vi "filter.delete.order.vi"(11 "filter.data in":T1 {"memory.command"."order.slot.value"."Quantity" format="%016x"; "memory.command"."order.slot.value"."OrderId" format="%016x"; "memory.command"."ticker.slot.value"."Symbol" format="%016x"; "Scratch"."OrderId" format="%016x"}) -> (3 "filter.data out":T1 {"memory.command"."order.slot.value"."Quantity" format="%016x"; "memory.command"."order.slot.value"."OrderId" format="%016x"; "memory.command"."ticker.slot.value"."Symbol" format="%016x"; "Scratch"."OrderId" format="%016x"})   [LabVIEW 2022 SP3]
uses:
  filter.data.ctl
  filter.states.ctl
  filter.debug.ctl
  filter.debug.slot.ctl
  filter.data.scratch.ctl
  common/orderbook.command.ctl
  common/orderbook.command.type.ctl
  filter.memory.command.ctl
  ticker.slot.ctl
  order.slot.ctl
  filter.getstate.ctl
  filter.getstate.slot.ctl
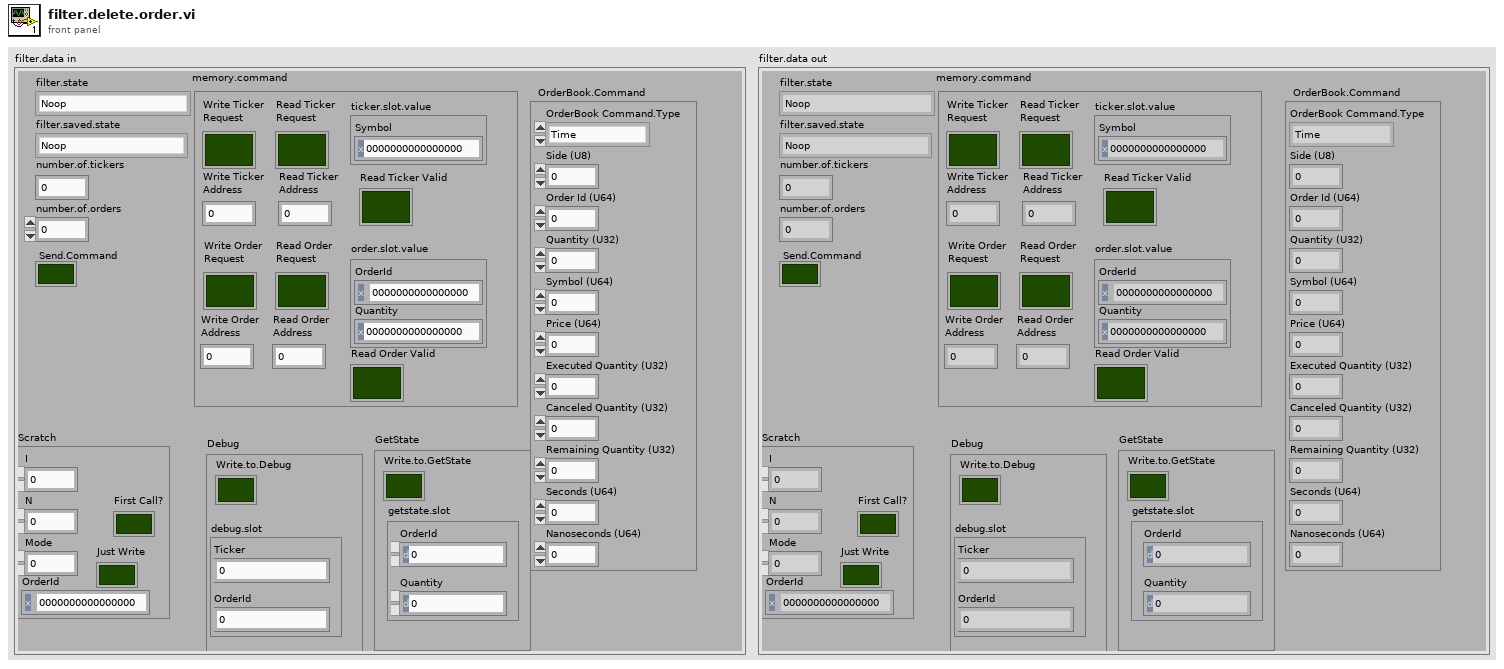
[diagram p1: front panel]
types:
  T1 = typedef "filter.data.ctl" = cluster{"filter.state":T2, "Debug":T3, "number.of.tickers":u32, "number.of.orders":u32, "filter.saved.state":T2, "Scratch":T5, "OrderBook.Command":T6, "Send.Command":bool, "memory.command":T8, "GetState":T11}
  T2 = typedef "filter.states.ctl" = enum16{"Noop", "Reset", "Debug", "Configuration", "Get.State", "Wait.for.Command", "Filter.Add", "Filter.Other", "Insert.Order", "Delete Order"}
  T3 = typedef "filter.debug.ctl" = cluster{"Write.to.Debug":bool, "debug.slot":T4}
  T4 = typedef "filter.debug.slot.ctl" = cluster{"Ticker":u64, "OrderId":u64}
  T5 = typedef "filter.data.scratch.ctl" = cluster{"I":u32, "N":u32, "Mode":u32, "OrderId":u64, "First Call?":bool, "Just Write":bool}
  T6 = typedef "orderbook.command.ctl" = cluster{"OrderBook Command.Type":T7, "Side (U8)":u8, "Order Id (U64)":u64, "Quantity (U32)":u32, "Symbol (U64)":u64, "Price (U64)":u64, "Executed Quantity (U32)":u32, "Canceled Quantity (U32)":u32, "Remaining Quantity (U32)":u32, "Seconds (U64)":u64, "Nanoseconds (U64)":u64}
  T7 = typedef "orderbook.command.type.ctl" = enum16{"Time", "AddOrder", "OrderExecuted", "OrderExecutedAtPrice", "ReduceSize", "ModifyOrder", "DeleteOrder", "Get.State", "Get.All.Orders", "Get.Top"}
  T8 = typedef "filter.memory.command.ctl" = cluster{"ticker.slot.value":T9, "order.slot.value":T10, "Write Ticker\nAddress":u32, "Write Ticker\nRequest":bool, "Read Ticker\nRequest":bool, "Read Ticker\nAddress":u32, "Read Ticker Valid":bool, "Write Order\nAddress":u32, "Write Order\nRequest":bool, "Read Order\nRequest":bool, "Read Order\nAddress":u32, "Read Order Valid":bool}
  T9 = typedef "ticker.slot.ctl" = cluster{"Symbol":u64}
  T10 = typedef "order.slot.ctl" = cluster{"OrderId":u64, "Quantity":u64}
  T11 = typedef "filter.getstate.ctl" = cluster{"Write.to.GetState":bool, "getstate.slot":T12}
  T12 = typedef "filter.getstate.slot.ctl" = cluster{"OrderId":u64, "Quantity":u64}
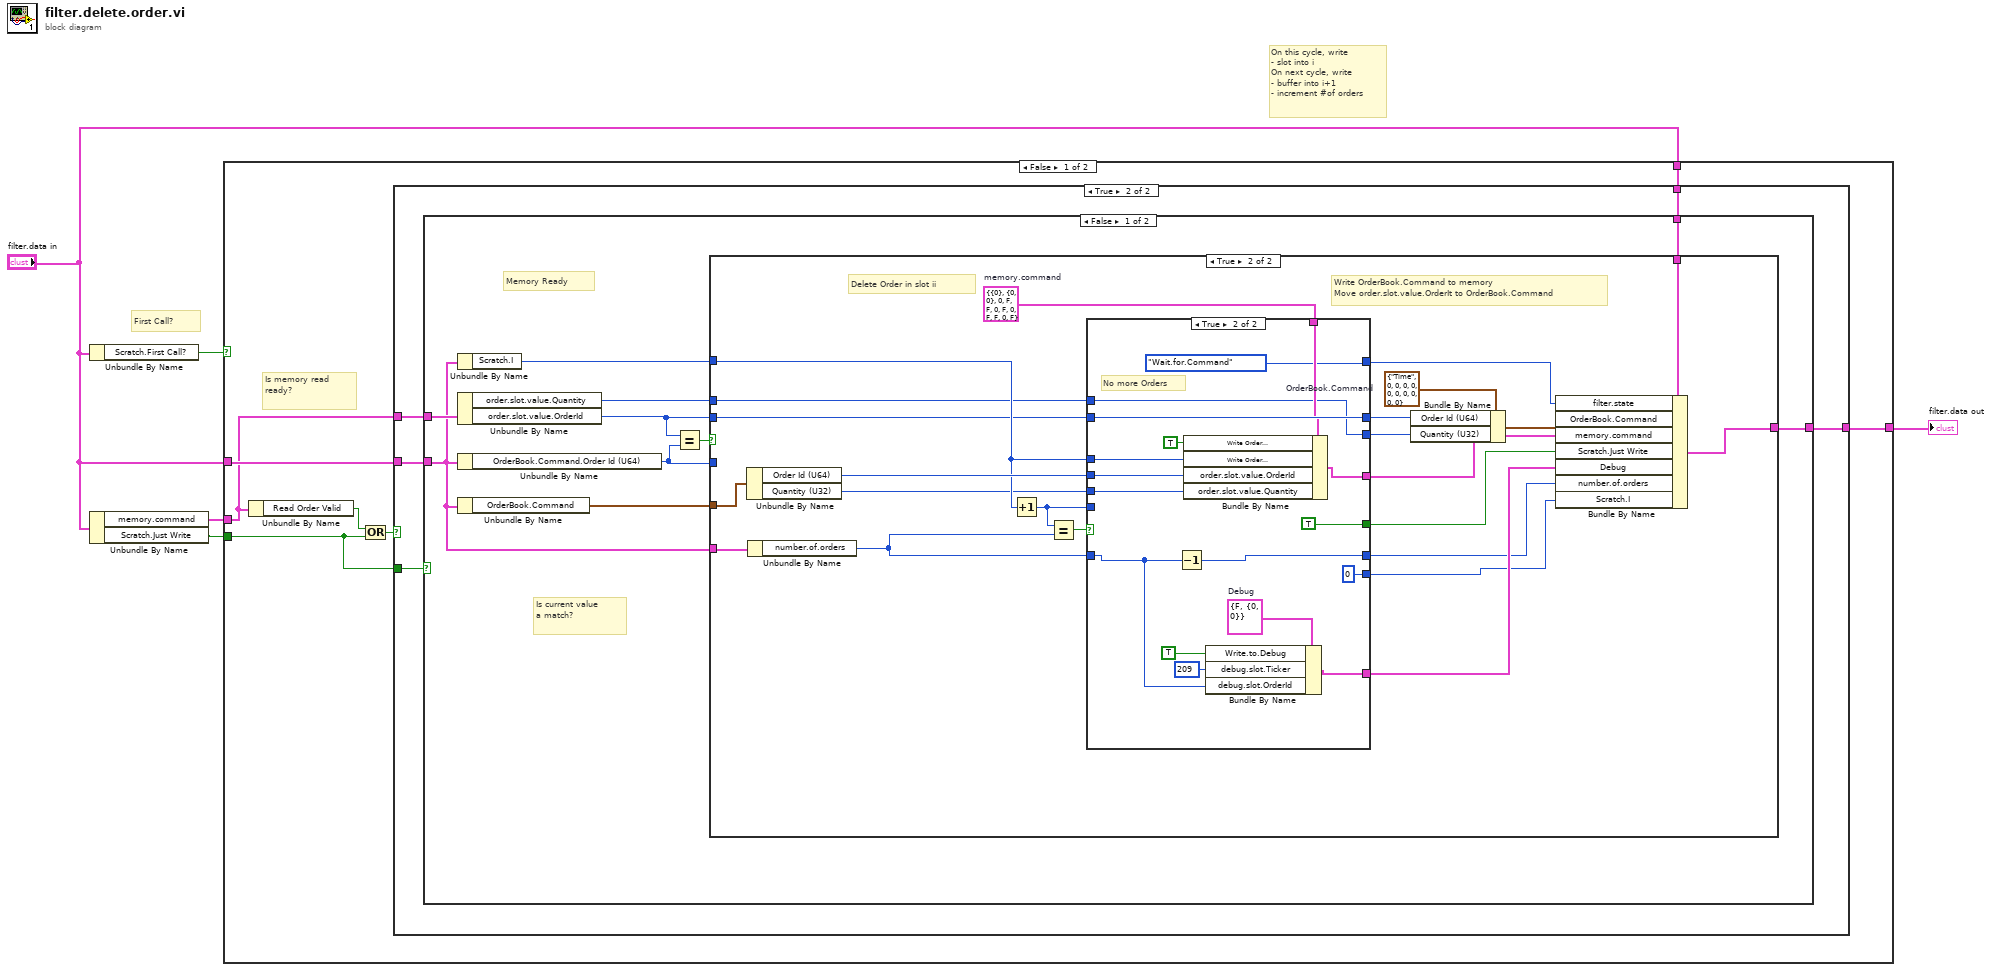
[diagram p0: block diagram]
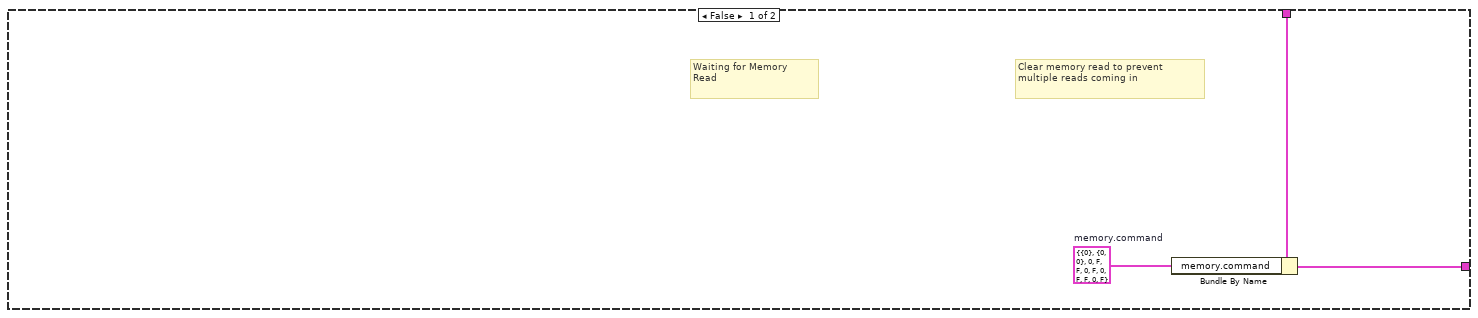
[diagram p2: hidden frame]
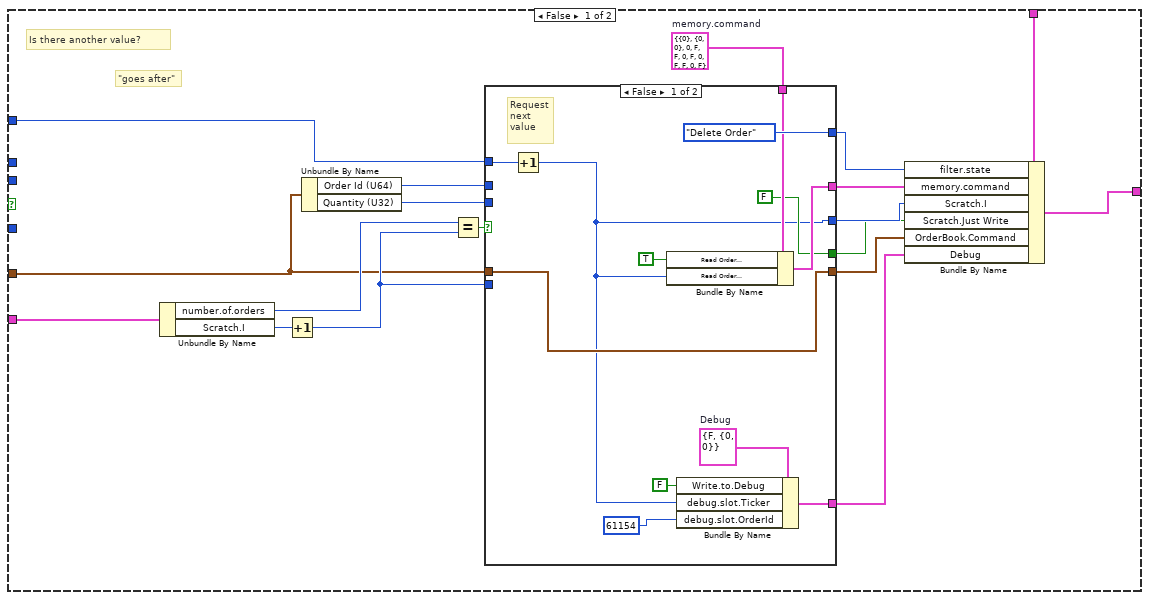
[diagram p3: hidden frame]
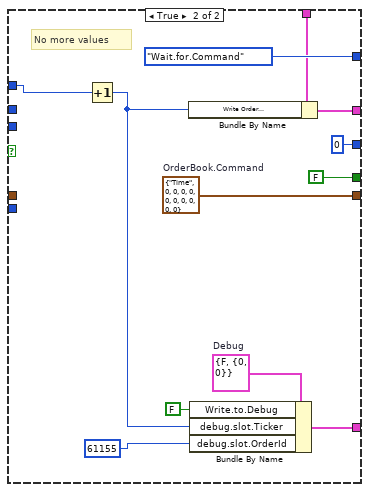
[diagram p4: hidden frame]
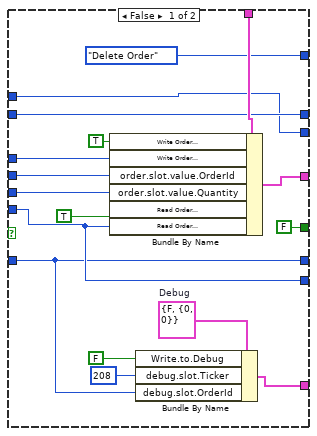
[diagram p5: hidden frame]
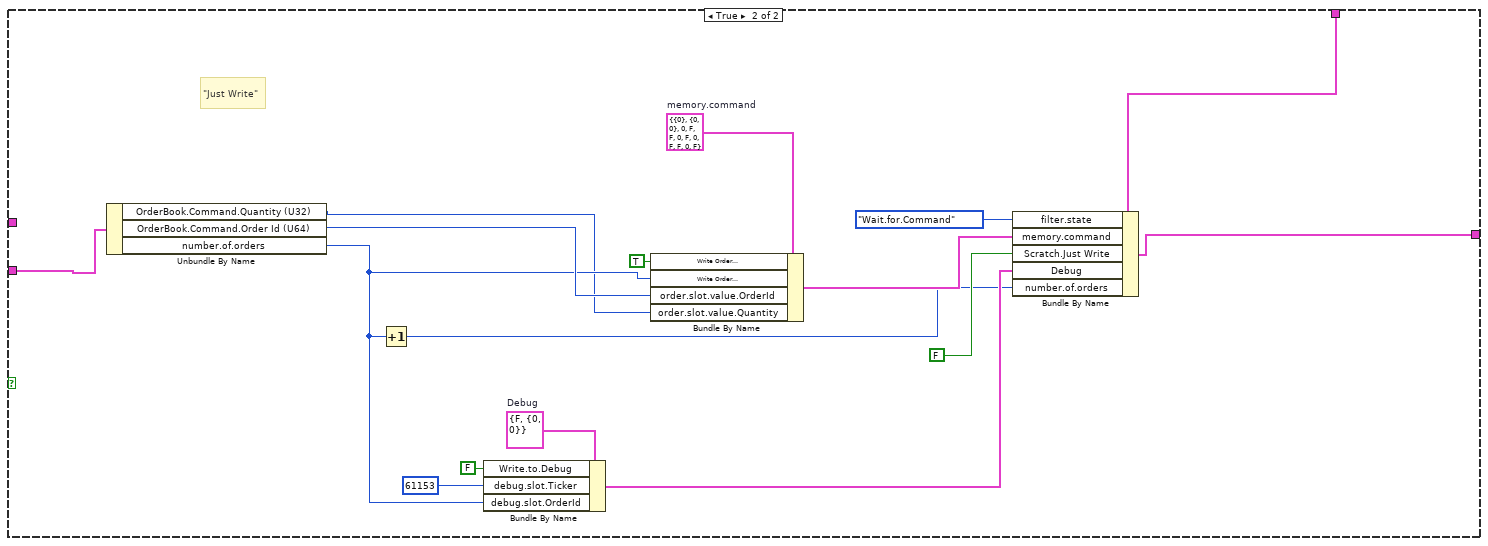
[diagram p6: hidden frame]
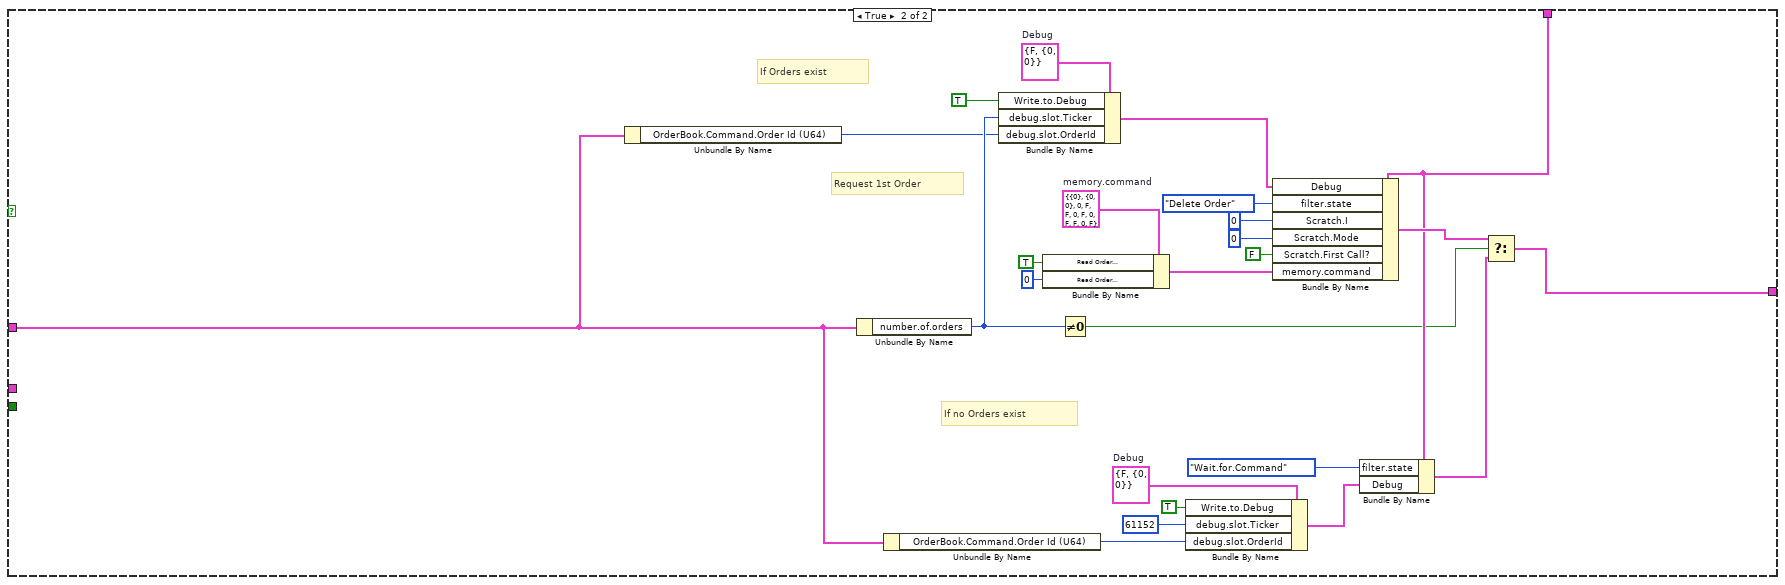
[diagram p7: hidden frame]
diagram:
  # "On this cycle, write\n- slot into i\nOn next cycle, write\n- buffer into i+1\n- increment #of orders"
  # "First Call?"
  n1 = Unbundle By Name("filter.data in") -> ("Scratch.First Call?"=w2:bool)
  n2 = Unbundle By Name("filter.data in") -> ("memory.command"=w4:T8, "Scratch.Just Write"=w1:bool)
  n3 = case shown="False" w2 {
    tunnel: "filter.data in" -> [w11 w159]
    tunnel: [w12 w163] -> w3
    tunnel: w4 -> [w9 _]
    tunnel: "filter.data in" -> [w10 w153]
    tunnel: w1 -> [w6 _]
    frame False {
      # "Is memory read\nready?"
      n4 = Unbundle By Name(w9) -> ("Read Order Valid"=w8:bool)
      n5 = Or(x=w8, y=w6) -> (x .or. y?=w7:bool)
      n6 = case shown="True" w7 {
        tunnel: [w13 w18] -> w12
        tunnel: w11 -> [w15 w19]
        tunnel: w10 -> [_ w17]
        tunnel: w9 -> [_ w20]
        tunnel: w6 -> [_ w16]
        frame False {
          w14 = T8 {"ticker.slot.value"={"Symbol"=0}, "order.slot.value"={"OrderId"=0, "Quantity"=0}, "Write Ticker\nAddress"=0, "Write Ticker\nRequest"=FALSE, "Read Ticker\nRequest"=FALSE, "Read Ticker\nAddress"=0, "Read Ticker Valid"=FALSE, "Write Order\nAddress"=0, "Write Order\nRequest"=FALSE, "Read Order\nRequest"=FALSE, "Read Order\nAddress"=0, "Read Order Valid"=FALSE}  # memory.command
          # "Clear memory read to prevent\nmultiple reads coming in"
          # "Waiting for Memory\nRead"
          n7 = Bundle By Name(cluster=w15, "memory.command"=w14) -> (w13:T1)
        }
        frame True {
          n8 = case shown="False" w16 {
            tunnel: w20 -> [w30 _]
            tunnel: w19 -> [w28 w141]
            tunnel: [w27 w140] -> w18
            tunnel: w17 -> [w23 w138]
            frame False {
              # "Is current value\na match?"
              # "Memory Ready"
              n9 = Unbundle By Name(w23) -> ("Scratch.I"=w22:u32)
              n10 = Unbundle By Name(w30) -> ("order.slot.value.Quantity"=w21:u64, "order.slot.value.OrderId"=w25:u64)
              n11 = Unbundle By Name(w23) -> ("OrderBook.Command.Order Id (U64)"=w24:u64)
              n12 = Unbundle By Name(w23) -> ("OrderBook.Command"=w26:T6)
              n13 = Equal?(x=w25, y=w24) -> (x = y?=w29:bool)
              n14 = case shown="True" w29 {
                tunnel: w28 -> [w47 w95]
                tunnel: [w48 w94] -> w27
                tunnel: w26 -> [w33 w89]
                tunnel: w23 -> [w46 w86]
                tunnel: w25 -> [_ w81]
                tunnel: w22 -> [w38 w87]
                tunnel: w24 -> [_ _]
                tunnel: w21 -> [_ w74]
                frame False {
                  w40 = T8 {"ticker.slot.value"={"Symbol"=0}, "order.slot.value"={"OrderId"=0, "Quantity"=0}, "Write Ticker\nAddress"=0, "Write Ticker\nRequest"=FALSE, "Read Ticker\nRequest"=FALSE, "Read Ticker\nAddress"=0, "Read Ticker Valid"=FALSE, "Write Order\nAddress"=0, "Write Order\nRequest"=FALSE, "Read Order\nRequest"=FALSE, "Read Order\nAddress"=0, "Read Order Valid"=FALSE}  # memory.command
                  # "\"goes after\""
                  # "Is there another value?"
                  n15 = Unbundle By Name(w46) -> ("number.of.orders"=w37:u32, "Scratch.I"=w45:u32)
                  n16 = Increment(x=w45) -> (x+1=w42:u32)
                  n17 = Unbundle By Name(w33) -> ("Order Id (U64)"=w39:u64, "Quantity (U32)"=w31:u32)
                  n18 = Equal?(x=w37, y=w42) -> (x = y?=w43:bool)
                  n19 = case shown="False" w43 {
                    tunnel: [w60 w70] -> w44
                    tunnel: w42 -> [_ _]
                    tunnel: [filter.states."Delete Order" ("filter.state") filter.states."Wait.for.Command" ("filter.state")] -> w41
                    tunnel: w40 -> [w57 w71]
                    tunnel: w39 -> [_ _]
                    tunnel: w38 -> [w50 w69]
                    tunnel: [w49 u32 0] -> w36
                    tunnel: [FALSE ("Scratch.Just Write") FALSE ("Scratch.Just Write")] -> w35
                    tunnel: [w55 w66] -> w34
                    tunnel: w33 -> [w55 _]
                    tunnel: [w53 w64] -> w32
                    tunnel: w31 -> [_ _]
                    frame False {
                      w54 = T3 {"Write.to.Debug"=FALSE, "debug.slot"={"Ticker"=0, "OrderId"=0}}  # Debug
                      # "Request\nnext\nvalue"
                      n20 = Increment(x=w50) -> (x+1=w49:u32)
                      n21 = Bundle By Name(cluster=w57, "Read Order\nRequest"=TRUE ("Read.Request"), "Read Order\nAddress"=w49) -> (w60:T8)
                      n22 = Bundle By Name(cluster=w54, "Write.to.Debug"=FALSE, "debug.slot.Ticker"=w49, "debug.slot.OrderId"=u64 61154) -> (w53:T3)
                    }
                    frame True {
                      w65 = T3 {"Write.to.Debug"=FALSE, "debug.slot"={"Ticker"=0, "OrderId"=0}}  # Debug
                      w66 = T6 {"OrderBook Command.Type"=enum."Time", "Side (U8)"=0, "Order Id (U64)"=0, "Quantity (U32)"=0, "Symbol (U64)"=0, "Price (U64)"=0, "Executed Quantity (U32)"=0, "Canceled Quantity (U32)"=0, "Remaining Quantity (U32)"=0, "Seconds (U64)"=0, "Nanoseconds (U64)"=0}  # OrderBook.Command
                      # "No more values"
                      n23 = Increment(x=w69) -> (x+1=w61:u32)
                      n24 = Bundle By Name(cluster=w71, "Write Order\nAddress"=w61) -> (w70:T8)
                      n25 = Bundle By Name(cluster=w65, "Write.to.Debug"=FALSE, "debug.slot.Ticker"=w61, "debug.slot.OrderId"=u64 61155) -> (w64:T3)
                    }
                  }
                  n26 = Bundle By Name(cluster=w47, "filter.state"=w41, "memory.command"=w44, "Scratch.I"=w36, "Scratch.Just Write"=w35, "OrderBook.Command"=w34, "Debug"=w32) -> (w48:T1)
                }
                frame True {
                  w92 = T6 {"OrderBook Command.Type"=enum."Time", "Side (U8)"=0, "Order Id (U64)"=0, "Quantity (U32)"=0, "Symbol (U64)"=0, "Price (U64)"=0, "Executed Quantity (U32)"=0, "Canceled Quantity (U32)"=0, "Remaining Quantity (U32)"=0, "Seconds (U64)"=0, "Nanoseconds (U64)"=0}  # OrderBook.Command
                  w91 = T8 {"ticker.slot.value"={"Symbol"=0}, "order.slot.value"={"OrderId"=0, "Quantity"=0}, "Write Ticker\nAddress"=0, "Write Ticker\nRequest"=FALSE, "Read Ticker\nRequest"=FALSE, "Read Ticker\nAddress"=0, "Read Ticker Valid"=FALSE, "Write Order\nAddress"=0, "Write Order\nRequest"=FALSE, "Read Order\nRequest"=FALSE, "Read Order\nAddress"=0, "Read Order Valid"=FALSE}  # memory.command
                  # "Write OrderBook.Command to memory\nMove order.slot.value.OrderIt to OrderBook.Command"
                  # "Delete Order in slot ii"
                  n27 = Unbundle By Name(w89) -> ("Order Id (U64)"=w88:u64, "Quantity (U32)"=w76:u32)
                  n28 = Unbundle By Name(w86) -> ("number.of.orders"=w78:u32)
                  n29 = Increment(x=w87) -> (x+1=w85:u32)
                  n30 = Equal?(x=w85, y=w78) -> (x = y?=w84:bool)
                  n31 = case shown="True" w84 {
                    tunnel: w91 -> [w112 w128]
                    tunnel: [w111 w127] -> w90
                    tunnel: w88 -> [w110 w126]
                    tunnel: w87 -> [w107 w119]
                    tunnel: w85 -> [w100 _]
                    tunnel: [w106 w129] -> w83
                    tunnel: w81 -> [w106 w129]
                    tunnel: [FALSE ("Scratch.Just Write") TRUE ("Scratch.Just Write")] -> w82
                    tunnel: [w101 w120] -> w80
                    tunnel: [w97 w115] -> w79
                    tunnel: w78 -> [w97 w114]
                    tunnel: [w100 u32 0] -> w77
                    tunnel: w76 -> [w99 w117]
                    tunnel: [w98 w116] -> w75
                    tunnel: w74 -> [w98 w116]
                    tunnel: [filter.states."Delete Order" ("filter.state") filter.states."Wait.for.Command" ("filter.state")] -> w73
                    frame False {
                      w104 = T3 {"Write.to.Debug"=FALSE, "debug.slot"={"Ticker"=0, "OrderId"=0}}  # Debug
                      n32 = Bundle By Name(cluster=w112, "Write Order\nRequest"=TRUE ("Write Order\nRequest"), "Write Order\nAddress"=w107, "order.slot.value.OrderId"=w110, "order.slot.value.Quantity"=w99, "Read Order\nRequest"=TRUE ("Read Order\nRequest"), "Read Order\nAddress"=w100) -> (w111:T8)
                      n33 = Bundle By Name(cluster=w104, "Write.to.Debug"=FALSE, "debug.slot.Ticker"=u64 208, "debug.slot.OrderId"=w97) -> (w101:T3)
                    }
                    frame True {
                      w123 = T3 {"Write.to.Debug"=FALSE, "debug.slot"={"Ticker"=0, "OrderId"=0}}  # Debug
                      # "No more Orders"
                      n34 = Decrement(x=w114) -> (x-1=w115:u32)
                      n35 = Bundle By Name(cluster=w128, "Write Order\nRequest"=TRUE ("Write Order\nRequest"), "Write Order\nAddress"=w119, "order.slot.value.OrderId"=w126, "order.slot.value.Quantity"=w117) -> (w127:T8)
                      n36 = Bundle By Name(cluster=w123, "Write.to.Debug"=TRUE, "debug.slot.Ticker"=u64 209, "debug.slot.OrderId"=w114) -> (w120:T3)
                    }
                  }
                  n37 = Bundle By Name(cluster=w92, "Order Id (U64)"=w83, "Quantity (U32)"=w75) -> (w93:T6)
                  n38 = Bundle By Name(cluster=w95, "filter.state"=w73, "OrderBook.Command"=w93, "memory.command"=w90, "Scratch.Just Write"=w82, "Debug"=w80, "number.of.orders"=w79, "Scratch.I"=w77) -> (w94:T1)
                }
              }
            }
            frame True {
              w137 = T3 {"Write.to.Debug"=FALSE, "debug.slot"={"Ticker"=0, "OrderId"=0}}  # Debug
              w143 = T8 {"ticker.slot.value"={"Symbol"=0}, "order.slot.value"={"OrderId"=0, "Quantity"=0}, "Write Ticker\nAddress"=0, "Write Ticker\nRequest"=FALSE, "Read Ticker\nRequest"=FALSE, "Read Ticker\nAddress"=0, "Read Ticker Valid"=FALSE, "Write Order\nAddress"=0, "Write Order\nRequest"=FALSE, "Read Order\nRequest"=FALSE, "Read Order\nAddress"=0, "Read Order Valid"=FALSE}  # memory.command
              # "\"Just Write\""
              n39 = Unbundle By Name(w138) -> ("OrderBook.Command.Quantity (U32)"=w130:u32, "OrderBook.Command.Order Id (U64)"=w134:u64, "number.of.orders"=w131:u32)
              n40 = Increment(x=w131) -> (x+1=w133:u32)
              n41 = Bundle By Name(cluster=w137, "Write.to.Debug"=FALSE, "debug.slot.Ticker"=u64 61153 ("debug.slot.OrderId"), "debug.slot.OrderId"=w131) -> (w135:T3)
              n42 = Bundle By Name(cluster=w143, "Write Order\nRequest"=TRUE ("Write Order\nRequest"), "Write Order\nAddress"=w131, "order.slot.value.OrderId"=w134, "order.slot.value.Quantity"=w130) -> (w139:T8)
              n43 = Bundle By Name(cluster=w141, "filter.state"=filter.states."Wait.for.Command", "memory.command"=w139, "Scratch.Just Write"=FALSE, "Debug"=w135, "number.of.orders"=w133) -> (w140:T1)
            }
          }
        }
      }
    }
    frame True {
      w151 = T3 {"Write.to.Debug"=FALSE, "debug.slot"={"Ticker"=0, "OrderId"=0}}  # Debug
      w157 = T3 {"Write.to.Debug"=FALSE, "debug.slot"={"Ticker"=0, "OrderId"=0}}  # Debug
      w169 = T8 {"ticker.slot.value"={"Symbol"=0}, "order.slot.value"={"OrderId"=0, "Quantity"=0}, "Write Ticker\nAddress"=0, "Write Ticker\nRequest"=FALSE, "Read Ticker\nRequest"=FALSE, "Read Ticker\nAddress"=0, "Read Ticker Valid"=FALSE, "Write Order\nAddress"=0, "Write Order\nRequest"=FALSE, "Read Order\nRequest"=FALSE, "Read Order\nAddress"=0, "Read Order Valid"=FALSE}  # memory.command
      # "If Orders exist"
      # "If no Orders exist"
      # "Request 1st Order"
      n44 = Unbundle By Name(w153) -> ("OrderBook.Command.Order Id (U64)"=w152:u64)
      n45 = Unbundle By Name(w153) -> ("number.of.orders"=w154:u32)
      n46 = Unbundle By Name(w153) -> ("OrderBook.Command.Order Id (U64)"=w149:u64)
      n47 = Bundle By Name(cluster=w157, "Write.to.Debug"=TRUE, "debug.slot.Ticker"=w154, "debug.slot.OrderId"=w152) -> (w155:T3)
      n48 = Bundle By Name(cluster=w169, "Read Order\nRequest"=TRUE ("Read.Request"), "Read Order\nAddress"=u32 0 ("Read Order\nAddress")) -> (w164:T8)
      n49 = Not Equal To 0?(x=w154) -> (x != 0?=w148:bool)
      n50 = Bundle By Name(cluster=w151, "Write.to.Debug"=TRUE, "debug.slot.Ticker"=u64 61152, "debug.slot.OrderId"=w149) -> (w146:T3)
      n51 = Bundle By Name(cluster=w159, "Debug"=w155, "filter.state"=filter.states."Delete Order", "Scratch.I"=u32 0, "Scratch.Mode"=u32 0, "Scratch.First Call?"=FALSE, "memory.command"=w164) -> (w162:T1)
      n52 = Bundle By Name(cluster=w159, "filter.state"=filter.states."Wait.for.Command", "Debug"=w146) -> (w160:T1)
      n53 = Select(t=w162, s=w148, f=w160) -> (s? t:f=w163:T1)
    }
  }
  "filter.data out" <- w3
